vi "map_data_func_global.vi"(7 "map_select":enum16{"up", "down", "same"}(ring), 8 "error in (no error)":errorcluster, 9 "write_map":bool, 10 "clear_map_array":bool, 11 "new_map":T1) -> (0 "error out":errorcluster, 1 "current_map":i32, 2 "maps_stored":i32, 3 "map_out":T1)   [LabVIEW 2015]
uses:
  map_data.ctl
  <vilib>/Utility/miscctls.llb/LVOffsetAndMultiplierTypeDef.ctl
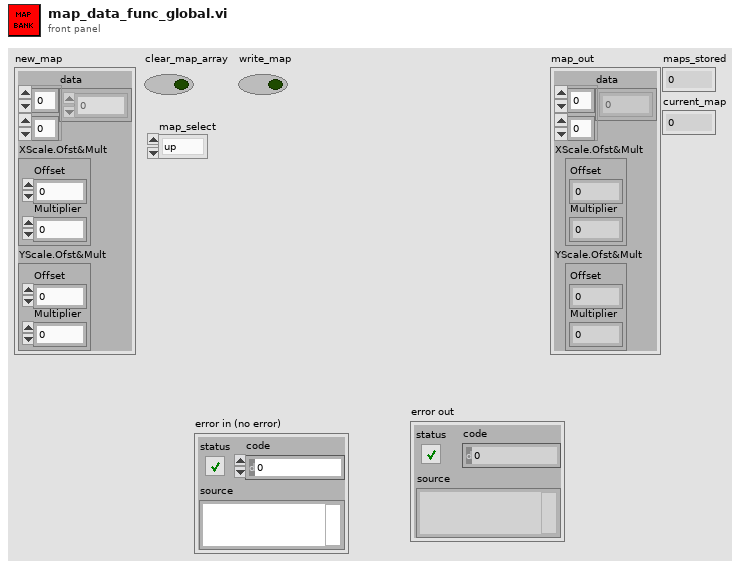
[diagram p1: front panel]
types:
  T1 = typedef "map_data.ctl" = cluster{"data":dbl[][], "XScale.Ofst&Mult":T2, "YScale.Ofst&Mult":T2}
  T2 = typedef "LVOffsetAndMultiplierTypeDef.ctl" = cluster{"Offset":dbl, "Multiplier":dbl}
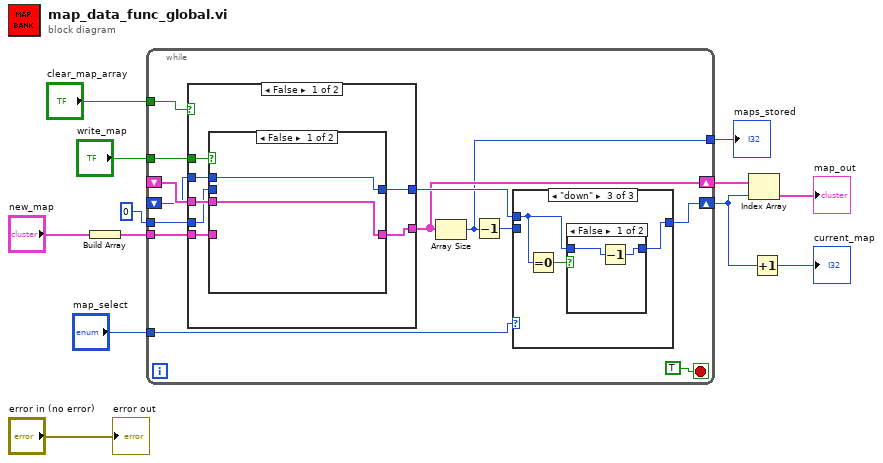
[diagram p0: block diagram]
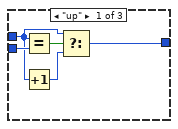
[diagram p2: hidden frame]
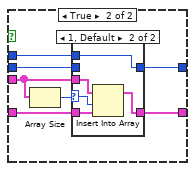
[diagram p5: hidden frame]
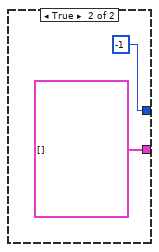
[diagram p7: hidden frame]
diagram:
  n1 = Build Array("new_map") -> (w11:T1[])
  n2 = while {
    shift-right: [w15] -> w10
    shift-left: _ -> [w24]
    tunnel: w11 -> [w25]
    tunnel: "clear_map_array" -> [w22]
    shift-right: [w18] -> w2
    shift-left: _ -> [w17]
    tunnel: 0 -> [w21]
    tunnel: "map_select" -> [w20]
    tunnel: "write_map" -> [w16]
    tunnel: [w13] -> w3
    stop <- TRUE stop-if-true
    n3 = case shown="False" w22 {
      tunnel: w25 -> [w44 _]
      tunnel: [w43 T1[] []] -> w15
      tunnel: w24 -> [w42 _]
      tunnel: w21 -> [w41 _]
      tunnel: [w40 -1] -> w19
      tunnel: w17 -> [w39 _]
      tunnel: w16 -> [w38 _]
      frame False {
        n4 = case shown="False" w38 {
          tunnel: w44 -> [_ w53]
          tunnel: [w46 w52] -> w43
          tunnel: w42 -> [w46 w51]
          tunnel: w41 -> [_ w49]
          tunnel: [w45 w48] -> w40
          tunnel: w39 -> [w45 w47]
          frame False {
          }
          frame True {
            n5 = Array Size(array=w51) -> (size(s)=w50:i32)
            n6 = case shown="1, Default" w50 {
              selector: w50 -> [_ w59]
              tunnel: w53 -> [w55 w58]
              tunnel: [w55 w57] -> w52
              tunnel: w51 -> [_ w60]
              tunnel: w49 -> [w54 _]
              tunnel: [w54 w56] -> w48
              tunnel: w47 -> [_ w56]
              frame 0 {
              }
              frame 1, Default {
                n7 = Insert Into Array(array=w60, index=w59, new element=w58) -> (w57:T1[])
              }
            }
          }
        }
      }
      frame True {
      }
    }
    n8 = Array Size(array=w15) -> (size(s)=w13:i32)
    n9 = Decrement(x=w13) -> (x-1=w14:i32)
    n10 = case shown="\"down\"" w20 {
      tunnel: w19 -> [w28 w31 w33]
      tunnel: [w26 w31 w32] -> w18
      tunnel: w14 -> [w30 _ _]
      frame "up" {
        n11 = Equal?(x=w28, y=w30) -> (x = y?=w29:bool)
        n12 = Increment(x=w28) -> (x+1=w27:i32)
        n13 = Select(t=w28, s=w29, f=w27) -> (s? t:f=w26:i32)
      }
      frame "same", Default {
      }
      frame "down" {
        n14 = Equal To 0?(x=w33) -> (x = 0?=w34:bool)
        n15 = case shown="False" w34 {
          tunnel: w33 -> [w36 w37]
          tunnel: [w35 w37] -> w32
          frame False {
            n16 = Decrement(x=w36) -> (x-1=w35:i32)
          }
          frame True {
          }
        }
      }
    }
  }
  "maps_stored" <- w3
  n17 = Index Array(array=w10, index=w2) -> (element=→"map_out":T1)
  n18 = Increment(x=w2) -> (x+1=→"current_map":i32)
  "error out" <- "error in (no error)"
